vi "Write Header to String Array.vi"(8 "error in (no error)":errorcluster, 11 "Header in":refnum<class "Header.lvclass">) -> (0 "error out":errorcluster, 3 "Header out":refnum<class "Header.lvclass">)   [LabVIEW 2018]
uses:
  Header.lvclass
  C:/Users/observer/Desktop/SPARC4_ACS/Simulated_Header/Simulated_Header.lvclass
panel:
  in  "Image Delays Settings":T1
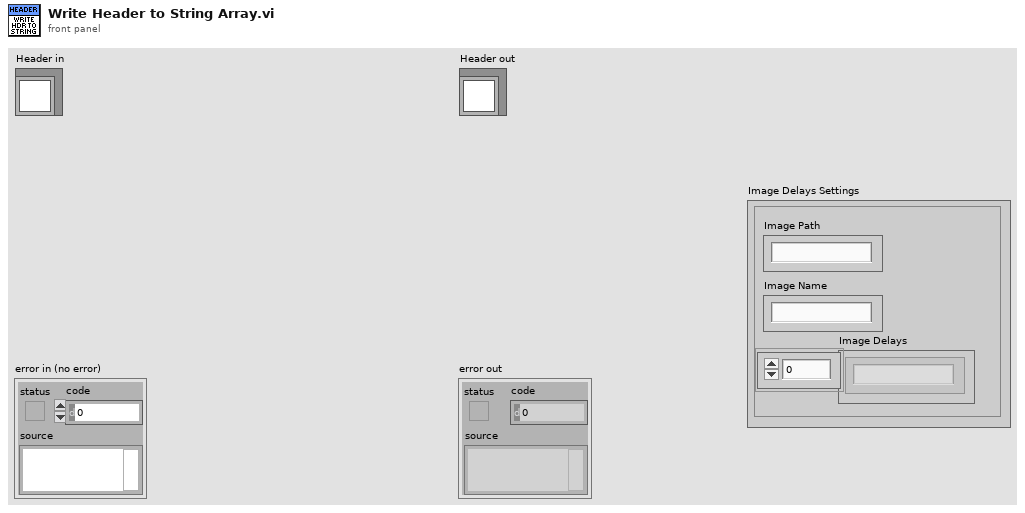
[diagram p1: front panel]
types:
  T1 = cluster{"Image Path":string, "Image Name":string, "Image Delays":string[]}
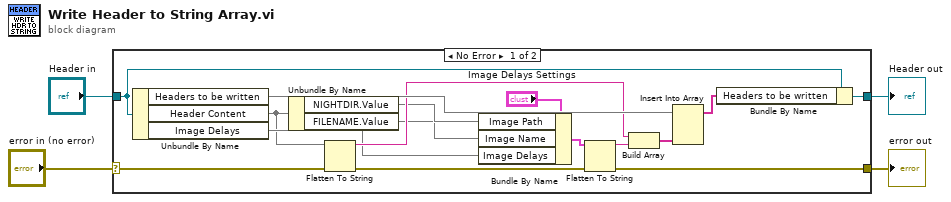
[diagram p0: block diagram]
diagram:
  n1 = case shown="No Error" "error in (no error)" {
    selector: "error in (no error)" -> [w20 w22]
    tunnel: [w11 w22] -> w3
    tunnel: [w17 w21] -> w1
    tunnel: "Header in" -> [w18 w21]
    frame No Error {
      n2 = Unbundle By Name(w18) -> ("Headers to be written"=w19, "Header Content"=w8, "Image Delays"=w9)
      n3 = Unbundle By Name(w8) -> ("NIGHTDIR.Value"=w7, "FILENAME.Value"=w6)
      n4 = Flatten To String(anything=w8, error in (no error)=w20) -> (data string=w15:string, error out=w12:errorcluster)  [unwired: 2 in, 1 out]
      n5 = Bundle By Name(cluster="Image Delays Settings", "Image Path"=w7, "Image Name"=w6, "Image Delays"=w9) -> (w5:T1)
      n6 = Flatten To String(anything=w5, error in (no error)=w12) -> (data string=w14:string, error out=w11:errorcluster)  [unwired: 2 in, 1 out]
      n7 = Build Array(w15, w14) -> (w13:string[])
      n8 = Insert Into Array(array=w19, new element=w13) -> (w16:string[])  [unwired: 2 in]
      n9 = Bundle By Name(cluster=w18, "Headers to be written"=w16) -> (w17:refnum<class "Header.lvclass">)
    }
    frame Error {
    }
  }
  "error out" <- w3
  "Header out" <- w1
